vi "通讯参数设置.vi"(4 "波特率":u32=19200) -> (2 "A设备簇":T1)   [LabVIEW 2020]
uses:
  <vilib>/NI/Modbus Library/API/Master/Modbus Master.lvclass
  <vilib>/NI/Modbus Library/API/Wrapper/Create Serial Master.vi
  <vilib>/NI/Modbus Library/API/Wrapper/API Main.lvlib
panel:
  out "信息显示":string
  in  "串口号":refnum<visa-resource-name>
  in  "ID站号":u8=1
  in  "校验位":u16(ring) items=["None", "Odd", "Even", "Mark", "Space"]
  in  "传输模式":enum16{"RTU", "ASCII"}(ring)
  in  "流控制":u16(ring) items=["None", "XON/XOFF", "RTS/CTS", "XON/XOFF & RTS/CTS", "DTR/DSR", "XON/XOFF & DTR/DSR"]
  in  "连接成功":bool
  out "A启用?":bool
  out "A实体":refnum<class "Modbus Master.lvclass">
  # "信息显示"
  # "通讯参数"
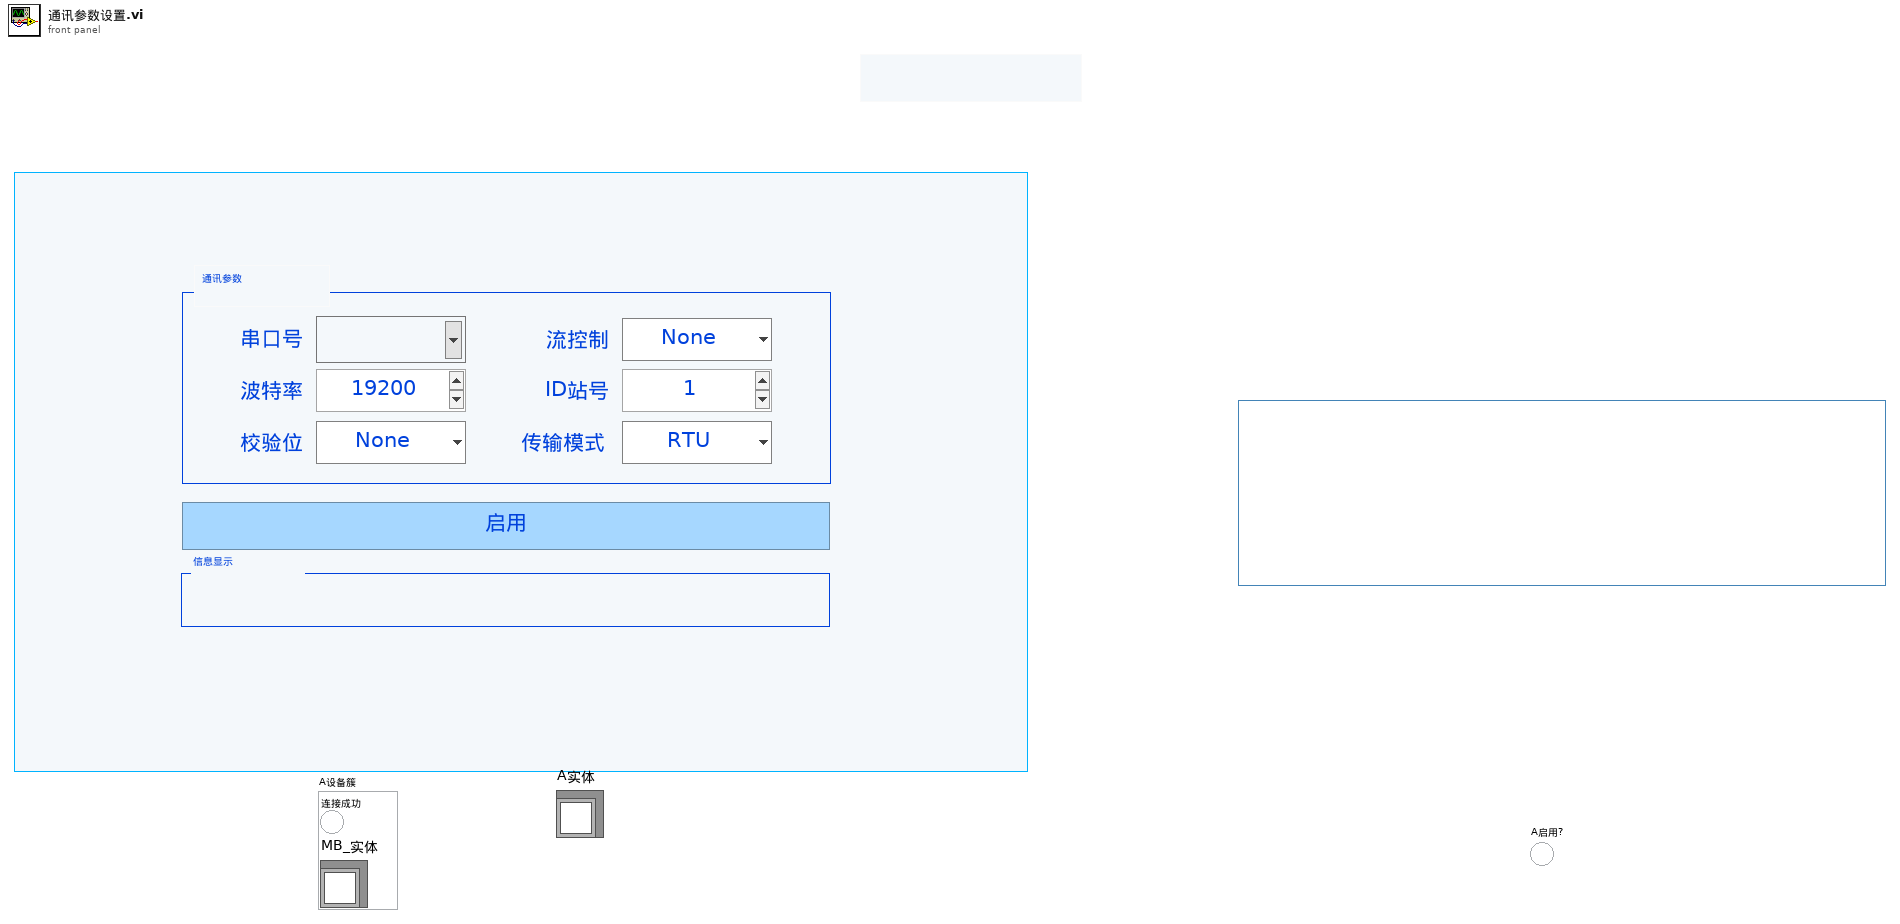
[diagram p1: front panel]
types:
  T1 = cluster{"连接成功":bool, "MB_实体":refnum<class "Modbus Master.lvclass">}
  T2 = cluster{"连接成功":bool, "A实体":refnum<class "Modbus Master.lvclass">}
  T3 = enum8{"Enabled", "Disabled", "Disabled and Grayed Out"}
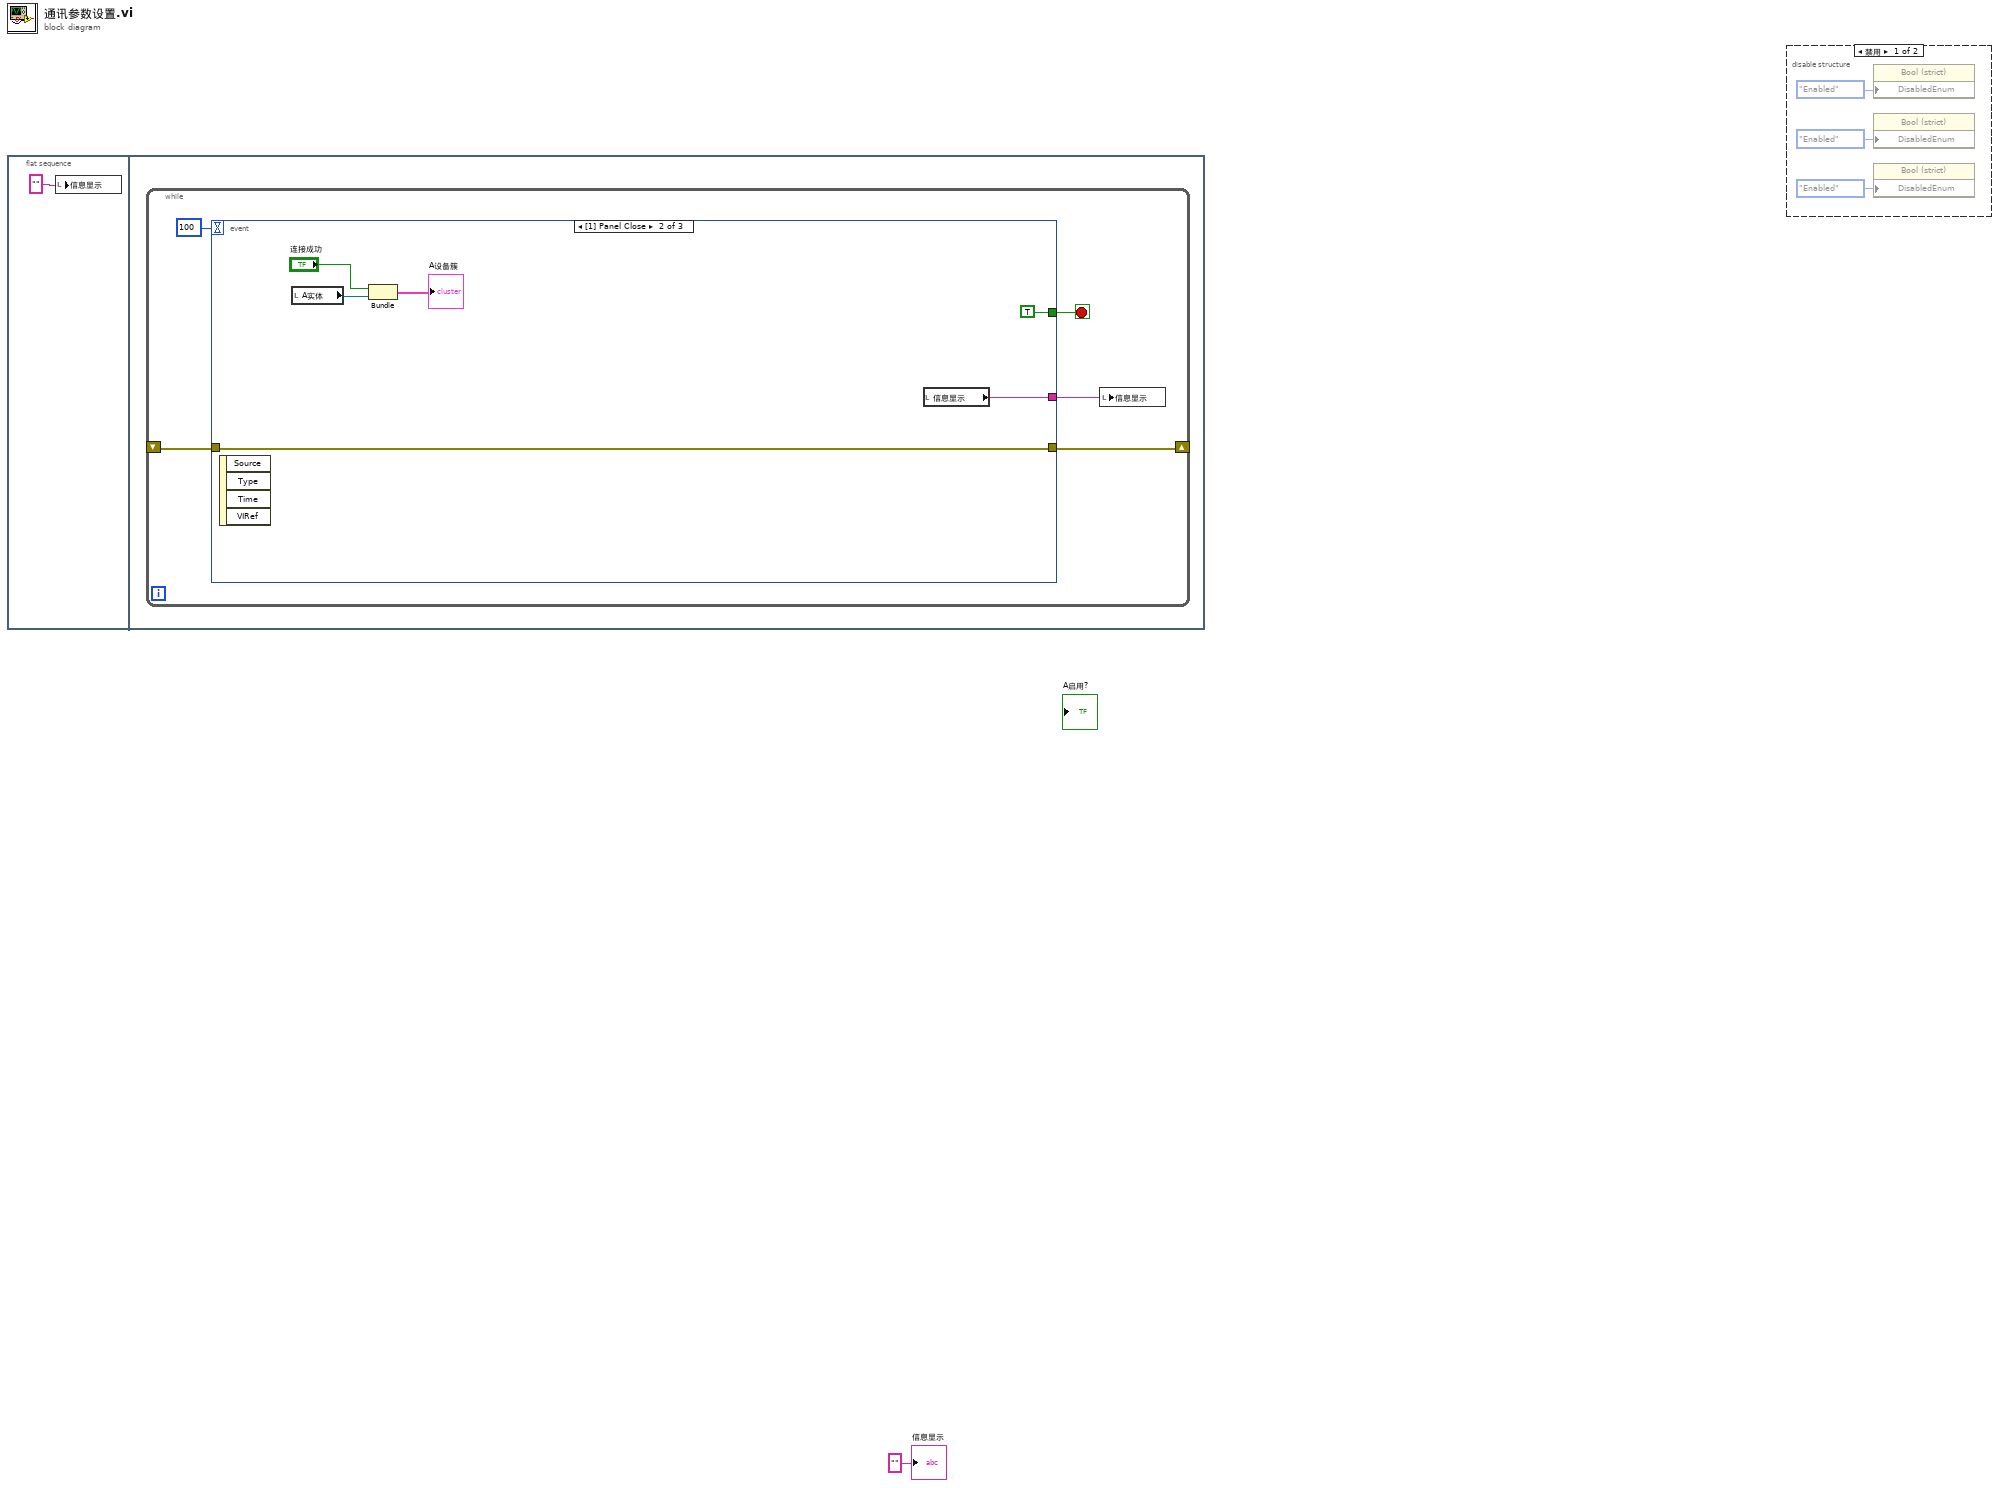
[diagram p0: block diagram]
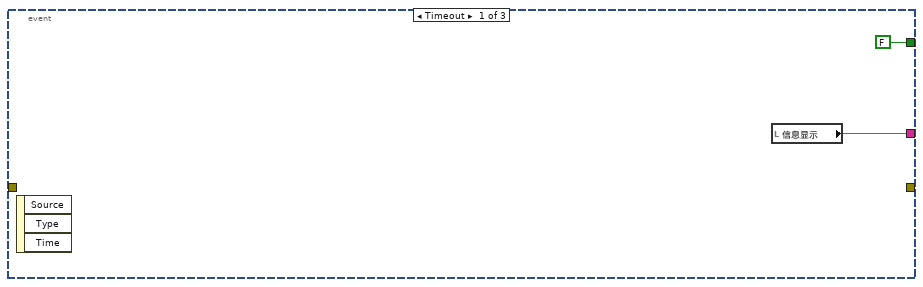
[diagram p2: hidden frame]
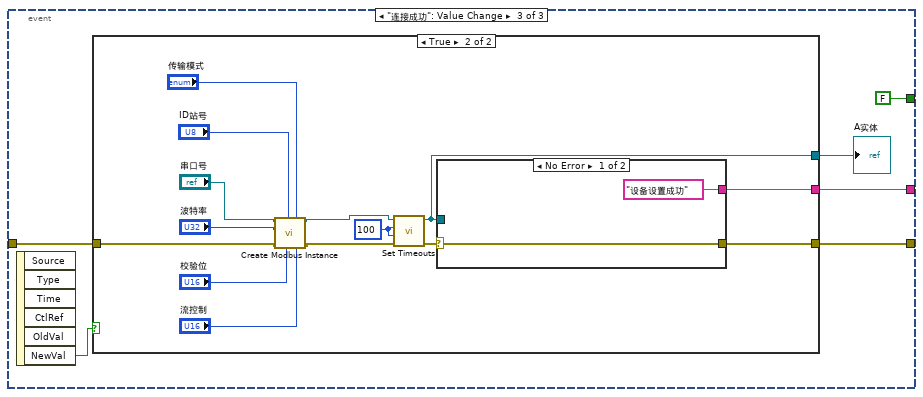
[diagram p3: hidden frame]
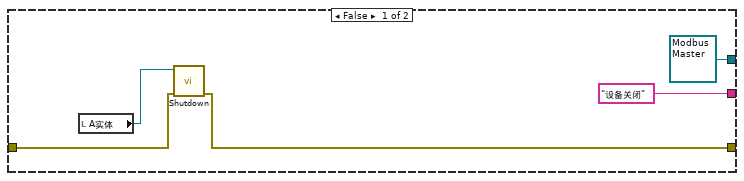
[diagram p4: hidden frame]
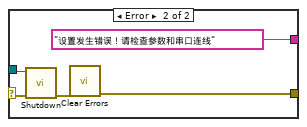
[diagram p5: hidden frame]
diagram:
  n1 = flat-sequence {
    frame #0 {
      n2 = local write "信息显示"("" ("信息显示")) -> ()
    }
    frame #1 {
      n3 = while {
        shift-right: [w4] -> _
        shift-left: _ -> [w5]
        stop <- w3 stop-if-true
        n4 = event shown="[1] Panel Close" {
          selector: _ -> [_ _ _]
          dyn-events: _ -> [_ _ _]
          timeout: 100 -> [_ _ _]
          tunnel: [w8 w13 w21] -> w7
          tunnel: w5 -> [_ w15 w18]
          tunnel: [_ w15 w20] -> w4
          tunnel: [FALSE ("Discard?") TRUE ("Discard?") FALSE ("Discard?")] -> w3
          event Timeout {
            n5 = event-data() -> ()  [unwired: 1 in, 3 out]
            n6 = local read "信息显示"() -> (w8:string)
          }
          event Panel Close {
            n7 = event-data() -> ()  [unwired: 1 in, 4 out]
            n8 = local read "A实体"() -> (w12:refnum<class "Modbus Master.lvclass">)
            n9 = Bundle("连接成功"="连接成功", "A实体"=w12) -> (→"A设备簇":T2)  [unwired: 1 in]
            n10 = local read "信息显示"() -> (w13:string)
          }
          event "连接成功": Value Change {
            n11 = event-data() -> ("NewVal"=w17:bool)  [unwired: 1 in, 5 out]
            n12 = case shown="True" w17 {
              tunnel: ["设备关闭" ("消息") w40] -> w21
              tunnel: [w23 w39] -> w20
              tunnel: w18 -> [w24 w31]
              tunnel: [refnum<class "Modbus Master.lvclass"> refnum ("serial master instance") w36] -> w16
              frame False {
                n13 = local read "A实体"() -> (w22:refnum<class "Modbus Master.lvclass">)
                n14 = call-dynamic "Shutdown.vi"("error in"=w24, "Modbus master in"=w22) -> ("error out"=w23:errorcluster)  [unwired: 9 in]
              }
              frame True {
                w38 = 100 ("read operation timeout (ms)")
                n15 = call-poly <vilib>:"Create Modbus Instance.vi"("flow control (none)"="流控制", "serial type"="传输模式", "parity (even)"="校验位", "unit ID"="ID站号", "error in"=w31, "baud rate"="波特率", "VISA resource name"="串口号") -> ("error out"=w30:errorcluster, "serial master instance"=w29:refnum<class "Modbus Master.lvclass">)  [unwired: 3 in]
                n16 = call <vilib>:"Set Timeouts.vi"("error in"=w30, "write operation timeout"=w38, "read operation timeout"=w38, "Modbus master in"=w29) -> ("error out"=w37:errorcluster, "Modbus master out"=w36:refnum<class "Modbus Master.lvclass">)  [unwired: 6 in]
                n17 = case shown="No Error" w37 {
                  selector: w37 -> [w42 w44]
                  tunnel: [w42 w47] -> w39
                  tunnel: ["设备设置成功" ("消息") "设置发生错误！请检查参数和串口连线" ("消息")] -> w40
                  tunnel: w36 -> [_ w45]
                  frame No Error {
                  }
                  frame Error {
                    n18 = call-dynamic "Shutdown.vi"("error in"=w44, "Modbus master in"=w45) -> ("error out"=w43:errorcluster)  [unwired: 9 in]
                    n19 = call <vilib>:"Clear Errors.vi"("error in (no error)"=w43) -> ("error out"=w47:errorcluster)  [unwired: 5 in, 1 out]
                  }
                }
              }
            }
            "A实体" <- w16
          }
        }
        n20 = local write "信息显示"(w7) -> ()
      }
    }
  }
  n21 = disable-structure shown="禁用" {
    frame Disabled {
      n22 = property on="属性节点" class="Bool (strict)"("DisabledEnum"=T3."Enabled" ("禁用")) -> (reference=w53:refnum<vi>)  [unwired: 1 in, 2 out]
      n23 = property on="属性节点" class="Bool (strict)"("DisabledEnum"=T3."Enabled" ("禁用")) -> (reference=w52:refnum<vi>)  [unwired: 1 in, 2 out]
      n24 = property on="属性节点" class="Bool (strict)"("DisabledEnum"=T3."Enabled" ("禁用")) -> (reference=w51:refnum<vi>)  [unwired: 1 in, 2 out]
    }
    frame Enabled {
    }
  }
  "信息显示" <- "" ("信息显示")
